vi "CheckPiecesToScore.vi"() -> ()   [LabVIEW 2018]
uses:
  Framework/Robot Global Data.vi
panel:
  in  "PiecesScored":u16
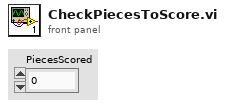
[diagram p1: front panel]
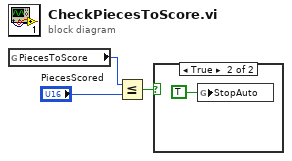
[diagram p0: block diagram]
diagram:
  n1 = global read "Robot Global Data.vi" "PiecesToScore"() -> (w3:u16)
  n2 = Less Or Equal?(x=w3, y="PiecesScored") -> (x <= y?=w1:bool)
  n3 = case shown="True" w1 {
    frame False {
    }
    frame True {
      n4 = global write "Robot Global Data.vi" "StopAuto"(TRUE ("StopAuto")) -> ()
    }
  }
